vi "DAQmx Read (Counter 1D Pulse Ticks 1Chan NSamp).vi"(0 "task/channels in":refnum<k21>, 7 "number of samples per channel":i32=-1, 9 "timeout":dbl=10.0 format="%0.2f", 11 "error in":errorcluster) -> (4 "task out":refnum<k21>, 6 "data":cluster{"high ticks":u32, "low ticks":u32}[](array[cluster]), 15 "error out":errorcluster)   [LabVIEW 2011]
doc: "Reads one or more pairs of pulse high and low tick counts from a counter input task."
uses:
  nilvaiu.dll
panel:
  # "sample #"
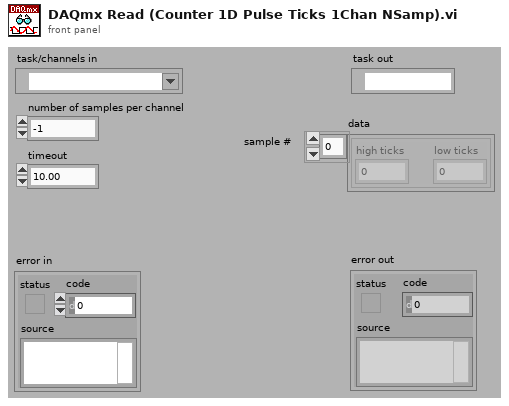
[diagram p1: front panel]
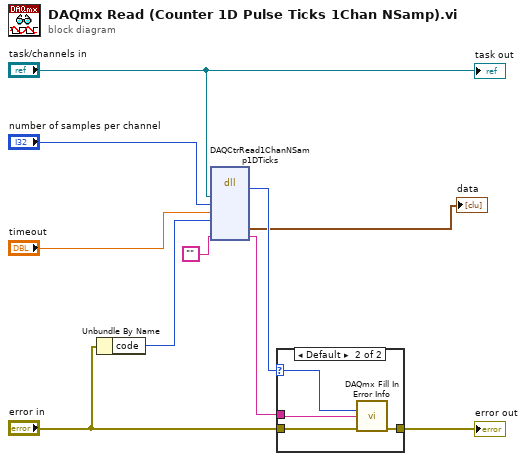
[diagram p0: block diagram]
diagram:
  n1 = Unbundle By Name("error in") -> ("code"=w2:i32)
  n2 = dll-call lib="nilvaiu.dll" fn="DAQCtrRead1ChanNSamp1DTicks"("taskID"="task/channels in", "numberOfSamples"="number of samples per channel", "timeout"="timeout", "incomingStatus"=w2, "extendedErrorInfo"="") -> ("return type"=w8:i32, "data"=→"data":cluster{"high ticks":u32, "low ticks":u32}[], "extendedErrorInfo"=w5:string)  [unwired: 7 in, 3 out]
  n3 = case shown="Default" w8 {
    selector: w8 -> [_ w13]
    tunnel: "error in" -> [w11 w15]
    tunnel: [w11 w14] -> w10
    tunnel: w5 -> [_ w12]
    frame 0 {
    }
    frame Default {
      n4 = call "DAQmx Fill In Error Info.vi"("status code"=w13, "extended error info"=w12, "error in"=w15) -> ("error out"=w14:errorcluster)  [unwired: 1 in, 11 out]
    }
  }
  "error out" <- w10
  "task out" <- "task/channels in"
